vi "test harness_FXP_K_times_X_single_axis.vi"(8 "error in (no error)":errorcluster, 11 "TestCase in":refnum<class "FXP_observer_TestCase.lvclass">) -> (0 "error out":errorcluster, 3 "TestCase out":refnum<class "FXP_observer_TestCase.lvclass">)   [LabVIEW 2017, in "FXP_observer_TestCase.lvclass"]
uses:
  FXP_observer_TestCase.lvclass
  <vilib>/rvi/DesktopExecutionNode/Execution/niFpgaDEN_Execute.vi
  <vilib>/rvi/DesktopExecutionNode/DesktopExecutionNode.xnode
  <vilib>/addons/_JKI Toolkits/VI Tester/TestCase.llb/TestCase.lvclass
  C:/Program Files (x86)/National Instruments/LabVIEW 2017/vi.lib/addons/_JKI Toolkits/VI Tester/TestCase.llb/TestCase.lvclass
panel:
  out "K*x":dbl
  in  "xerr":fxp<+/-,32,5>[](array[numeric])=[1.0, 2.0, 5.0, 2.0, 0.0, 0.0, 0.0, 0.0, 0.0, 0.0, 0.0, 0.0, 0.0, 0.0, 0.0, 0.0, 0.0, 0.0, 0.0, 0.0, 0.0, 0.0, 0.0, 0.0, 0.0, 0.0, 0.0, 0.0, 0.0, 0.0, 0.0, 0.0, 0.0, 0.0, 0.0, 0.0, 0.0, 0.0, 0.0, 0.0, 0.0, 0.0, 0.0, 0.0, 0.0, 0.0, 0.0, 0.0]
  in  "NS + 2":u8=5
  out "K*x (expected)":dbl
  in  "K_lqr":fxp<+/-,32,5>[](array[numeric])=[10.0, 0.5, 0.20000000298023224, 0.20000000298023224, 0.29999999701976776, 2.0, 0.0, 0.0, 0.0, 0.0, 0.0, 0.0, 0.0, 0.0, 0.0, 0.0, 0.0, 0.0, 0.0, 0.0, 0.0, 0.0, 0.0, 0.0, 0.0, 0.0, 0.0, 0.0, 0.0, 0.0, 0.0, 0.0, 0.0, 0.0, 0.0, 0.0, 0.0, 0.0, 0.0, 0.0, 0.0, 0.0, 0.0, 0.0, 0.0, 0.0, 0.0, 0.0, 0.0, 0.0]
  in  "x":fxp<+/-,32,5>[](array[numeric])=[1.0, 2.0, 3.0, 2.0, 6.0, 8.0, 0.0, 0.0, 0.0, 0.0, 0.0, 0.0, 0.0, 0.0, 0.0, 0.0, 0.0, 0.0, 0.0, 0.0, 0.0, 0.0, 0.0, 0.0, 0.0, 0.0, 0.0, 0.0, 0.0, 0.0, 0.0, 0.0, 0.0, 0.0, 0.0, 0.0, 0.0, 0.0, 0.0, 0.0, 0.0, 0.0, 0.0, 0.0, 0.0, 0.0, 0.0, 0.0, 0.0, 0.0]
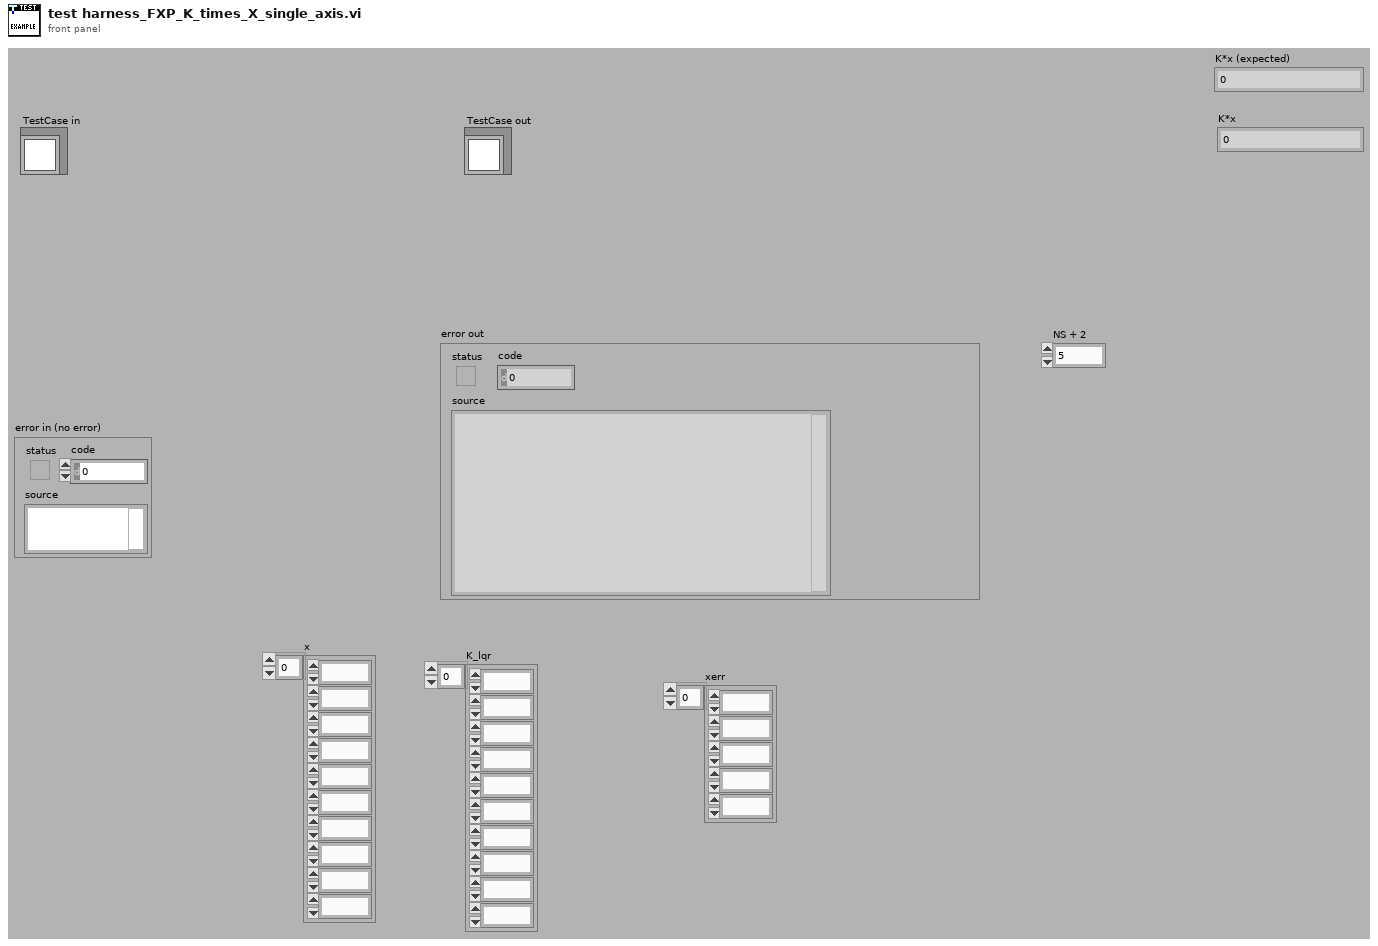
[diagram p1: front panel]
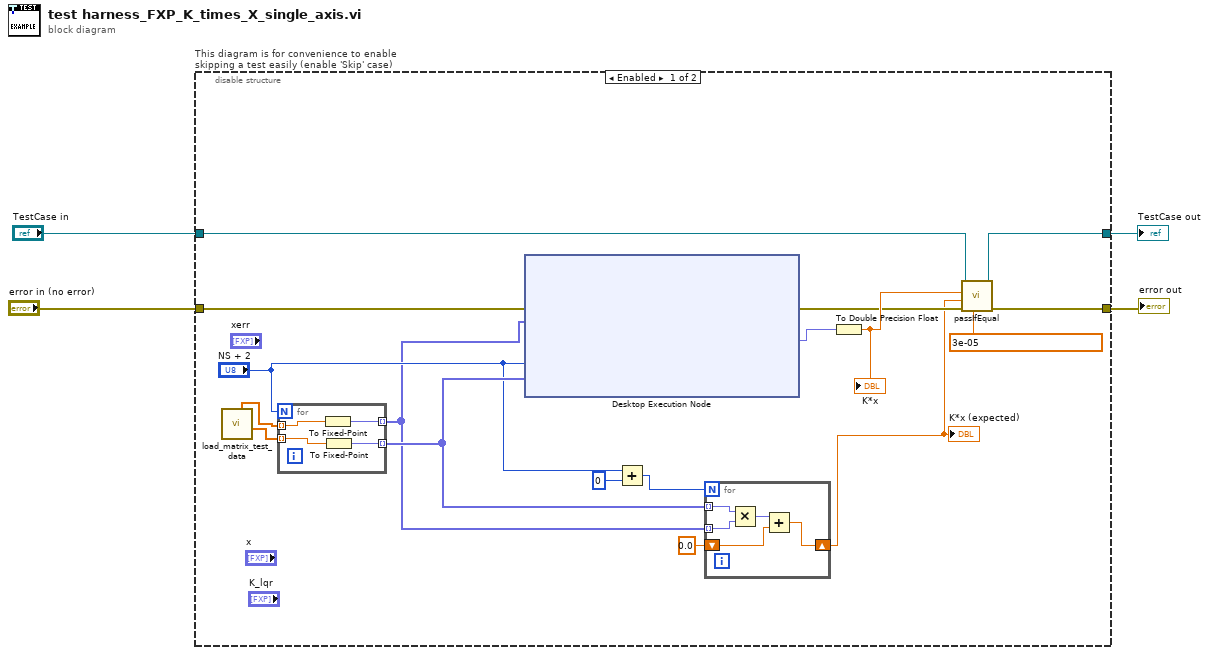
[diagram p0: block diagram]
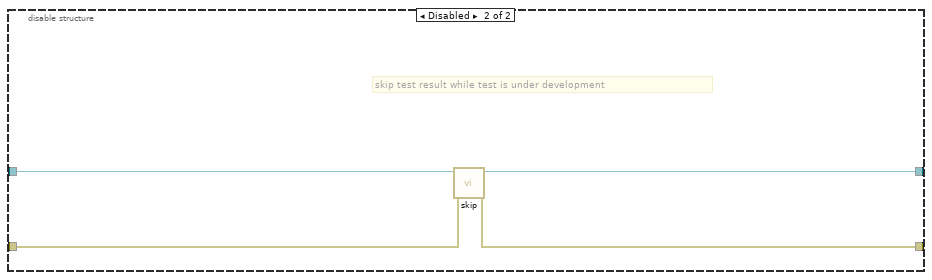
[diagram p2: hidden frame]
diagram:
  n1 = disable-structure "This diagram is for convenience to enable skipping a test easily (enable 'Skip' case)" shown="Enabled" {
    disable-tunnel: "TestCase in" -> [w21 w34]
    disable-tunnel: [w20 w32] -> w1
    disable-tunnel: [w19 w33] -> w3
    disable-tunnel: "error in (no error)" -> [w15 w31]
    frame Enabled {
      n2 = call "load_matrix_test_data.vi"() -> ("Kz"=w13:dbl[], "X_test"=w5:dbl[])  [unwired: 5 in, 5 out]
      n3 = for {
        N: "NS + 2" -> [_]
        tunnel: w13 -> [w30] mode=indexing
        tunnel: [w29] -> w12 mode=indexing
        tunnel: w5 -> [w28] mode=indexing
        tunnel: [w27] -> w6 mode=indexing
        n4 = To Fixed-Point(number=w28) -> (fixed-point=w27:fxp<+/-,32,6>)  [unwired: 1 in]
        n5 = To Fixed-Point(number=w30) -> (fixed-point=w29:fxp<+/-,32,15>)  [unwired: 1 in]
      }
      n6 = xnode "Desktop Execution Node"("Error In"=w15, "x_vec"=w6, "NS + 2"="NS + 2", "K_lqr"=w12) -> ("Error Out"=w16:errorcluster, "del u_x"=w18:fxp<+/-,64,15>)
      n7 = Add(x="NS + 2", y=i8 0) -> (x+y=w9:u8)
      n8 = for {
        N: w9 -> [_]
        tunnel: w12 -> [w25] mode=indexing
        tunnel: w6 -> [w24] mode=indexing
        shift-right: [w23] -> w10
        shift-left: 0.0 -> [w22]
        n9 = Multiply(x=w25, y=w24) -> (x*y=w26:fxp<+/-,64,21>)
        n10 = Add(x=w26, y=w22) -> (x+y=w23:dbl)
      }
      "K*x (expected)" <- w10
      n11 = To Double Precision Float(number=w18) -> (double precision float=w17:dbl)
      "K*x" <- w17
      n12 = call-dynamic "passIfEqual.vi"("delta (optional)"=3e-05 ("del u_x"), "error in (no error)"=w16, "y"=w10, "x"=w17, "TestCase in"=w21) -> ("error out"=w19:errorcluster, "TestCase out"=w20:refnum<class "FXP_observer_TestCase.lvclass">)  [unwired: 5 in]
    }
    frame Disabled {
      # "skip test result while test is under development"
      n13 = call <vilib>:"skip.vi"("error in (no error)"=w31, "TestCase in"=w34) -> ("error out"=w33:errorcluster, "TestCase out"=w32:refnum<class "FXP_observer_TestCase.lvclass">)  [unwired: 8 in]
    }
  }
  "error out" <- w3
  "TestCase out" <- w1
